vi "保持力判定.vi"(4 "最大力":dbl=4.0, 6 "最小力":dbl=3.0, 7 "Result":refnum<vi>, 8 "最大位移":dbl=4.0, 9 "最小位移":dbl=3.0, 10 "判定参数":T1={"保持力最大力"={"单位"="N", "下限"=3.0, "上限"=4.0}, "保持力位移监控"={"单位"="N", "下限"=3.0, "上限"=4.0}}, 11 "XY曲线":cluster{"X":dbl[], "Y":dbl[]}[](array[cluster])) -> (2 "判定项长度":i32, 3 "OK？":bool)   [LabVIEW 2020]
panel:
  out "Y":dbl[](array[numeric])
  out "转置的数组":string[][](array[string])
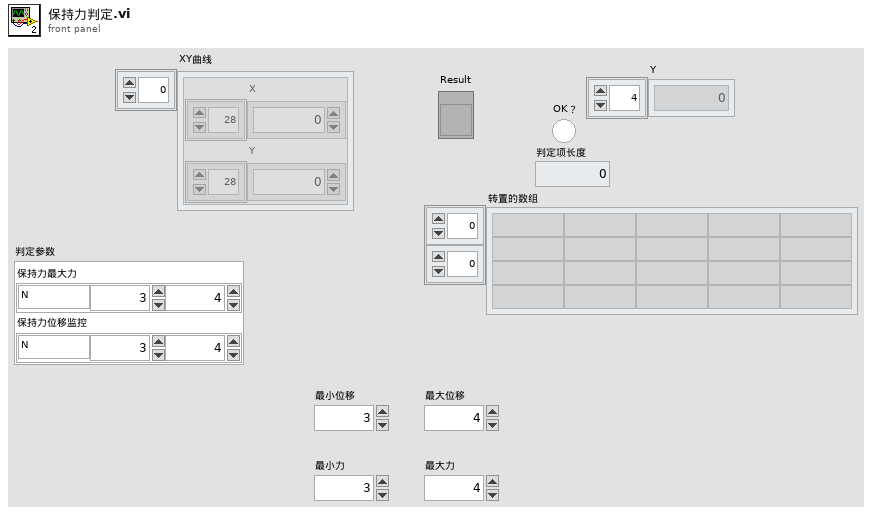
[diagram p1: front panel]
types:
  T1 = cluster{"保持力最大力":cluster{"单位":string, "下限":dbl, "上限":dbl}, "保持力位移监控":cluster{"单位":string, "下限":dbl, "上限":dbl}}
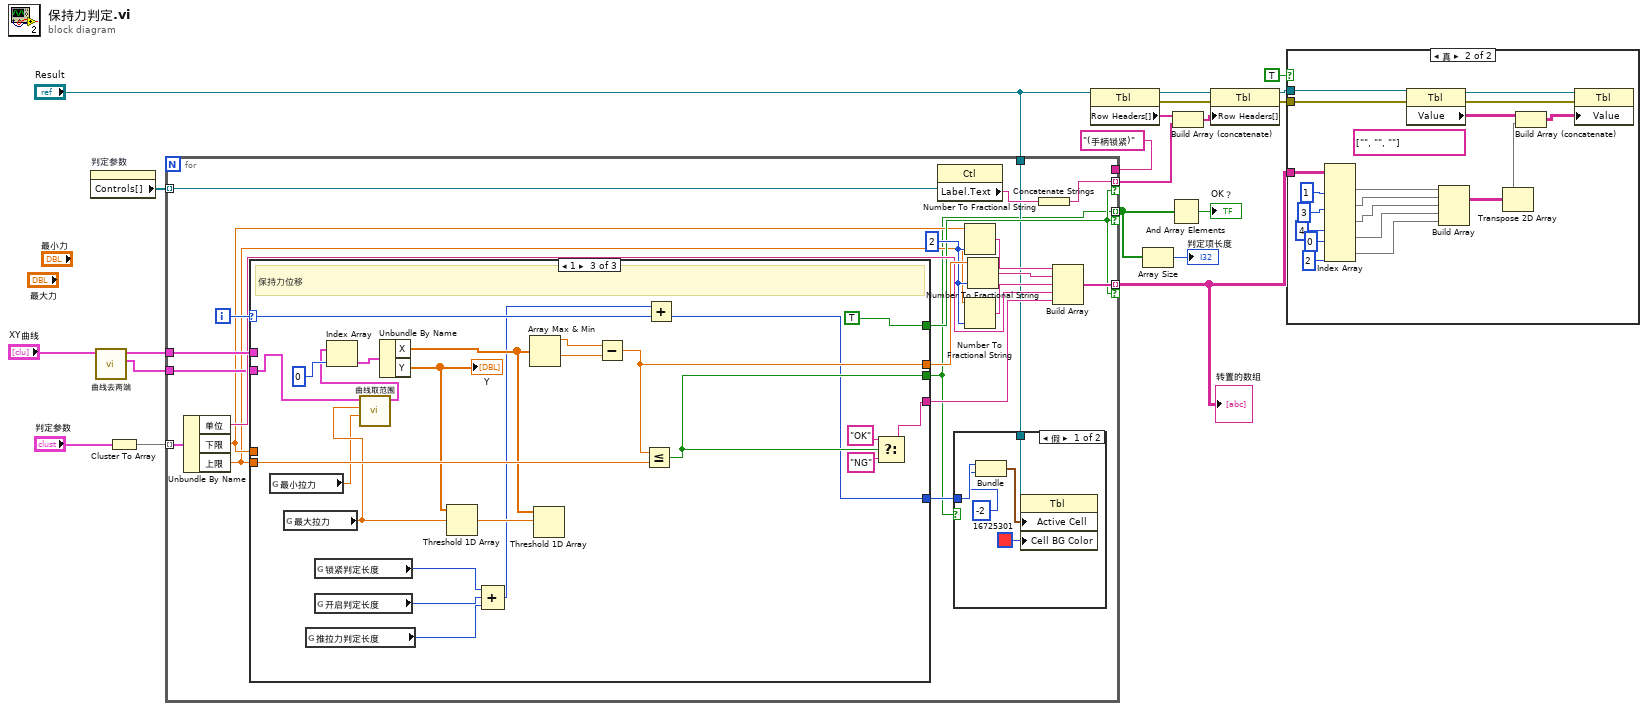
[diagram p0: block diagram]
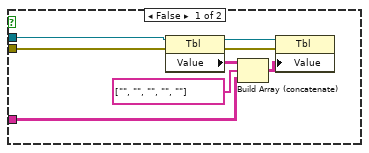
[diagram p2: hidden frame]
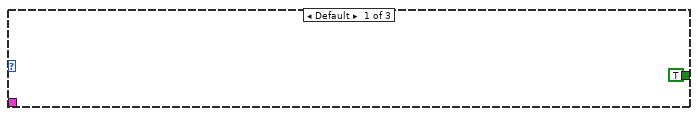
[diagram p4: hidden frame]
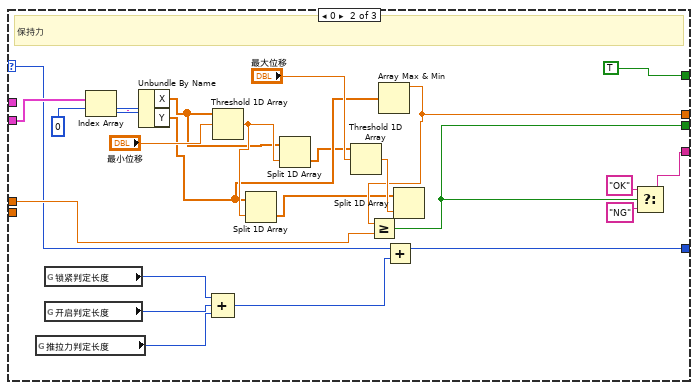
[diagram p5: hidden frame]
diagram:
  n1 = property on="判定参数" class="Clust (严格)"() -> ("Controls[]"=w12:refnum<vi>[])  [unwired: 2 in, 2 out]
  n2 = call "曲线去两端.vi"("曲线In"="XY曲线") -> ("启动曲线"=w5:cluster{"X":dbl[], "Y":dbl[]}[], "曲线Out"=w8:cluster{"X":dbl[], "Y":dbl[]}[])  [unwired: 9 in]
  n3 = Cluster To Array(cluster="判定参数") -> (array=w2:cluster{"单位":string, "下限":dbl, "上限":dbl}[])
  n4 = for {
    tunnel: w12 -> [w40] mode=indexing
    tunnel: w8 -> [w38]
    tunnel: [w21] -> w7 mode=indexing if=w29
    tunnel: [w31] -> w3 mode=indexing if=w29
    tunnel: [w25] -> w14 mode=indexing if=w29
    tunnel: w5 -> [w28]
    tunnel: "(手柄锁紧)" ("Label.Text") -> [_]
    tunnel: w2 -> [w24] mode=indexing
    tunnel: "Result" -> [w23]
    i -> [w41]
    w37 = i16 2 ("精度(6)")
    n5 = Unbundle By Name(w24) -> ("单位"=w32:string, "下限"=w27:dbl, "上限"=w26:dbl)
    n6 = case shown="1" w41 {
      selector: w41 -> [_ w53 w86]
      tunnel: [_ w60 w88] -> w39
      tunnel: w38 -> [_ _ _]
      tunnel: [_ w67 w91] -> w33
      tunnel: [_ w64 w89] -> w21
      tunnel: w27 -> [_ w65 _]
      tunnel: w26 -> [_ _ w87]
      tunnel: [TRUE TRUE TRUE] -> w29
      tunnel: w28 -> [_ w58 w76]
      tunnel: [_ w52 w85] -> w22
      frame Default {
      }
      frame 0 {
        # "保持力"
        n7 = global read "判定参数.vi" "推拉力判定长度"() -> (w49:i32)
        n8 = global read "判定参数.vi" "锁紧判定长度"() -> (w51:i32)
        n9 = global read "判定参数.vi" "开启判定长度"() -> (w50:i32)
        n10 = Index Array(array=w58, index=0 ("索引")) -> (element=w70:cluster{"X":dbl[], "Y":dbl[]})
        n11 = Unbundle By Name(w70) -> ("X"=w57:dbl[], "Y"=w55:dbl[])
        n12 = Compound Arithmetic op=ADD(w51, w50, w49) -> (w48:i32)
        n13 = Threshold 1D Array(2:"最小位移", 3:w57) -> (0:w59:dbl)  [unwired: 1 in]
        n14 = Split 1D Array(array=w55, index=w59) -> (second subarray=w56:dbl[])  [unwired: 1 out]
        n15 = Split 1D Array(array=w57, index=w59) -> (second subarray=w54:dbl[])  [unwired: 1 out]
        n16 = Threshold 1D Array(2:"最大位移", 3:w54) -> (0:w61:dbl)  [unwired: 1 in]
        n17 = Array Max & Min(array=w55) -> (max value=w60:dbl)  [unwired: 3 out]
        n18 = Greater Or Equal?(x=w60, y=w65) -> (x >= y?=w64:bool)
        n19 = Add(x=w53, y=w48) -> (x+y=w52:i32)
        n20 = Split 1D Array(array=w56, index=w61) -> ()  [unwired: 2 out]
        n21 = Select(t="OK", s=w64, f="NG") -> (s? t:f=w67:string)
      }
      frame 1 {
        # "保持力位移"
        n22 = global read "判定参数.vi" "最小拉力"() -> (w72:dbl)
        n23 = global read "判定参数.vi" "最大拉力"() -> (w75:dbl)
        n24 = global read "判定参数.vi" "推拉力判定长度"() -> (w78:i32)
        n25 = global read "判定参数.vi" "锁紧判定长度"() -> (w80:i32)
        n26 = global read "判定参数.vi" "开启判定长度"() -> (w79:i32)
        n27 = call "曲线取范围.vi"("下限"=w72, "上限"=w75, "曲线In"=w76) -> ("曲线Out"=w74:cluster{"X":dbl[], "Y":dbl[]}[])  [unwired: 8 in]
        n28 = Index Array(array=w74, index=0 ("索引")) -> (element=w94:cluster{"X":dbl[], "Y":dbl[]})
        n29 = Unbundle By Name(w94) -> ("X"=w82:dbl[], "Y"=w84:dbl[])
        "Y" <- w84
        n30 = Threshold 1D Array ("以阈值插值一维数组")(2:w75, 3:w84) -> (0:w83:dbl)  [unwired: 1 in]
        n31 = Compound Arithmetic op=ADD(w80, w79, w78) -> (w77:i32)
        n32 = Array Max & Min(array=w82) -> (max value=w73:dbl, min value=w81:dbl)  [unwired: 2 out]
        n33 = Threshold 1D Array(2:w83, 3:w82) -> ()  [unwired: 1 in, 1 out]
        n34 = Subtract(x=w73, y=w81) -> (x-y=w88:dbl)
        n35 = Less Or Equal?(x=w88, y=w87) -> (x <= y?=w89:bool)
        n36 = Add(x=w77, y=w86) -> (x+y=w85:i32)
        n37 = Select(t="OK", s=w89, f="NG") -> (s? t:f=w91:string)
      }
    }
    n38 = property class="Ctl"(reference=w40) -> ("Label.Text"=w30:string)  [unwired: 1 in, 2 out]
    n39 = case shown="假" w21 {
      tunnel: w23 -> [w46 _]
      tunnel: w22 -> [w44 _]
      frame False {
        n40 = Bundle(w44, "索引"=-2) -> (w42:cluster{i32, "索引":i32})  [unwired: 1 in]
        n41 = property class="Tbl"(reference=w46, "Active Cell"=w42, "Cell BG Color"=u32 16725301 ("活动单元格:单元格背景色")) -> ()  [unwired: 1 in, 2 out]
      }
      frame True {
      }
    }
    n42 = Number To Fractional String(number=w27, precision (6)=w37) -> (F-format string=w36:string)  [unwired: 2 in]
    n43 = Number To Fractional String(number=w26, precision (6)=w37) -> (F-format string=w34:string)  [unwired: 2 in]
    n44 = Number To Fractional String(number=w39, precision (6)=w37) -> (F-format string=w35:string)  [unwired: 2 in]
    n45 = Concatenate Strings(w30) -> (w25:string)
    n46 = Build Array(w36, w35, w34, w32, w33) -> (w31:string[])
  }
  "转置的数组" <- w3
  n47 = property class="Tbl"(reference="Result") -> (reference out=w16:refnum<vi>, error out=w19:errorcluster, "Row Headers[]"=w13:string[])  [unwired: 1 in]
  n48 = Array Size(array=w7) -> (size(s)=→"判定项长度":i32)
  n49 = And Array Elements(Boolean array=w7) -> (logical AND=→"OK？":bool)
  n50 = Build Array (concatenate)(w13, w14) -> (w15:string[])
  n51 = property class="Tbl"(reference=w16, error in=w19, "Row Headers[]"=w15) -> (reference out=w17:refnum<vi>, error out=w18:errorcluster)
  n52 = case shown="真" TRUE {
    tunnel: w18 -> [w101 w121]
    tunnel: w17 -> [w98 w118]
    tunnel: w3 -> [w97 w115]
    frame False {
      n53 = property class="Tbl"(reference=w98, error in=w101) -> (reference out=w99:refnum<vi>, error out=w100:errorcluster, "Value"=w102:string[][])
      n54 = Build Array (concatenate)(w102, string[] ["", "", "", "", ""], w97) -> (w103:string[][])
      n55 = property class="Tbl"(reference=w99, error in=w100, "Value"=w103) -> ()  [unwired: 2 out]
    }
    frame True {
      (unwired) string[] ["", "", ""]
      n56 = Index Array(array=w115, index (col) #1=1 ("禁用的索引 (列)"), index (col) #2=3 ("索引 (列)"), index (col) #3=4 ("索引 (列)"), index (col) #4=0 ("索引 (列)"), index (col) #5=2 ("索引 (列)")) -> (element #1=w110:string[], element #2=w109:string[], element #3=w108:string[], element #4=w107:string[], element #5=w106:string[])  [unwired: 5 in]
      n57 = property class="Tbl"(reference=w118, error in=w121) -> (reference out=w119:refnum<vi>, error out=w120:errorcluster, "Value"=w122:string[][])
      n58 = Build Array(w110, w109, w108, w107, w106) -> (w112:string[][])
      n59 = Transpose 2D Array ("二维数组转置")(2D array=w112) -> (transposed array=w104:string[][])
      n60 = Build Array (concatenate)(w122, w104) -> (w111:string[][])
      n61 = property class="Tbl"(reference=w119, error in=w120, "Value"=w111) -> ()  [unwired: 2 out]
    }
  }
